vi "Module Type.vi"(11 "Debug GUI Module in":refnum<class "Debug GUI Module.lvclass">) -> (2 "Module Type":string)   [LabVIEW 2020, in "VolatusGUI.lvlib" / "Debug GUI Module.lvclass"]
uses:
  Debug GUI Module.lvclass
  Debug GUI Module.lvclass/Debug GUI Module.ctl
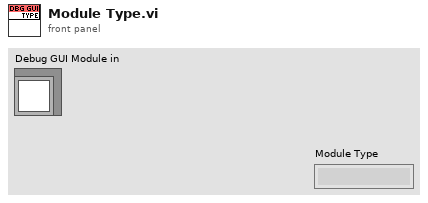
[diagram p1: front panel]
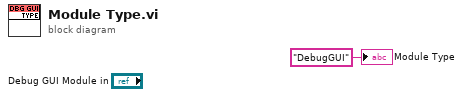
[diagram p0: block diagram]
diagram:
  "Module Type" <- "DebugGUI" ("Module Type")
